vi "XY Graph Savitzky-Golay Filter Plot.vi"(6 "Weight (none)":dbl[](array[numeric]), 8 "Error In":errorcluster, 9 "polynomial order  (3)":i32=3, 10 "side points (6)":i32=6, 11 "Plot in":cluster{"X Array":dbl[], "Y Array":dbl[]}) -> (0 "Error Out":errorcluster, 3 "Plot out":cluster{"X Array":dbl[], "Y Array":dbl[]})   [LabVIEW 2021, in "XY Graph Add-Ons.lvlib"]
uses:
  XY Graph Add-Ons.lvlib
  <vilib>/Analysis/3filter.llb/Savitzky-Golay Filter (DBL).vi
  <vilib>/Analysis/NI_AALBase.lvlib
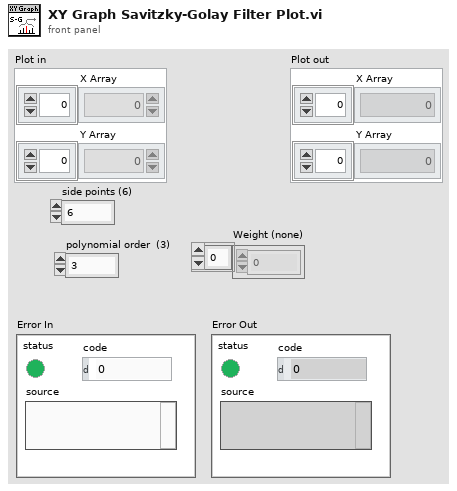
[diagram p1: front panel]
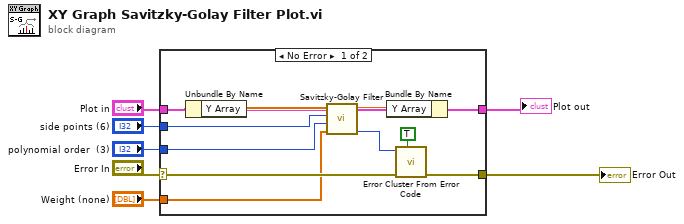
[diagram p0: block diagram]
diagram:
  n1 = case shown="No Error" "Error In" {
    selector: "Error In" -> [w13 w19]
    tunnel: "Plot in" -> [w17 w20]
    tunnel: [w15 w20] -> w6
    tunnel: [w12 w19] -> w4
    tunnel: "side points (6)" -> [w10 _]
    tunnel: "polynomial order  (3)" -> [w9 _]
    tunnel: "Weight (none)" -> [w8 _]
    frame No Error {
      n2 = Unbundle By Name(w17) -> ("Y Array"=w18:dbl[])
      n3 = call-poly <vilib>:"Savitzky-Golay Filter.vi"("Weight"=w8, "polynomial order"=w9, "side points"=w10, "X"=w18) -> ("error"=w14:i32, "Filtered X"=w16:dbl[])  [unwired: 6 in]
      n4 = Bundle By Name(cluster=w17, "Y Array"=w16) -> (w15:cluster{"X Array":dbl[], "Y Array":dbl[]})
      n5 = call <vilib>:"Error Cluster From Error Code.vi"("show call chain? (False)"=TRUE, "error in (no error)"=w13, "error code (0)"=w14) -> ("error out"=w12:errorcluster)  [unwired: 6 in]
    }
    frame Error {
    }
  }
  "Plot out" <- w6
  "Error Out" <- w4
